vi "Set Absoulute Target Position.vi"(0 "reference in":refnum<class "SmartMotor.lvclass">, 3 "Absoulute Target Position (Revolutions)":dbl, 5 "error in (no error)":errorcluster) -> (14 "reference out":refnum<class "SmartMotor.lvclass">, 19 "error out":errorcluster)   [LabVIEW 2017, in "SmartMotor.lvclass"]
uses:
  SmartMotor.lvclass
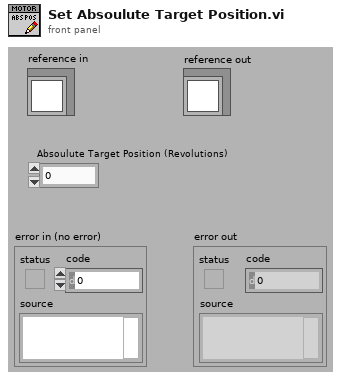
[diagram p1: front panel]
types:
  T1 = typedef "SmartMotor.lvclass/ObjectAttributes.ctl" = cluster{"SmartMotor Chain VISA Resource":refnum<visa-resource-name>, "SmartMotor Chain Address":i16, "Motor Absolute Position":i32, "Motor Relative Position":i32, "Motor Torque":i32, "Motor Voltage":i32, "Screwdriver Engaged":bool, "Screwdriver Torque Limit":i32, "Torque Monitor On/Off Status":bool, "Torque Monitor VI Reference":refnum<vi>, "Absolute Motor Torque (Filtered)":dbl, "SmartMotor Status":T2, "SmartMotor Error":T3}
  T2 = typedef "SmartMotor.lvclass/SmartMotor Status.ctl" = enum8{"Stopped", "Moving"}
  T3 = typedef "SmartMotor.lvclass/SmartMotor Error.ctl" = enum8{"None", "Read Error", "Low Voltage"}
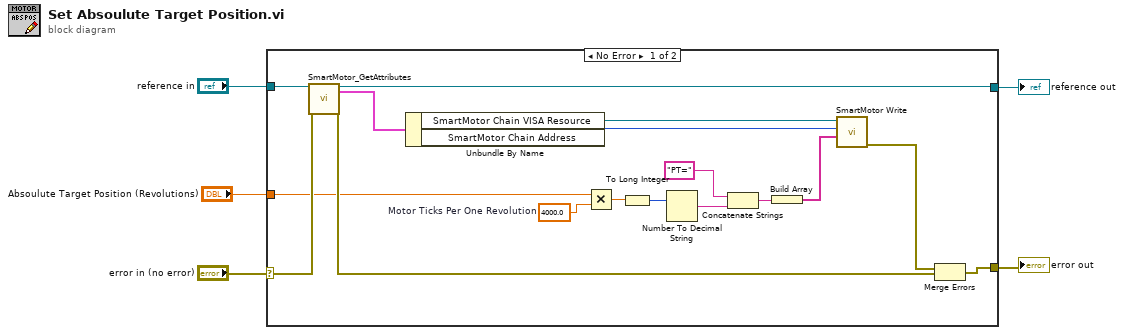
[diagram p0: block diagram]
diagram:
  n1 = case shown="No Error" "error in (no error)" {
    selector: "error in (no error)" -> [w21 w24]
    tunnel: [w19 w24] -> w4
    tunnel: [w20 w23] -> w2
    tunnel: "reference in" -> [w22 w23]
    tunnel: "Absoulute Target Position (Revolutions)" -> [w17 _]
    frame No Error {
      w15 = 4000.0  # Motor Ticks Per One Revolution
      n2 = call "SmartMotor_GetAttributes.vi"("reference in"=w22, "error in (no error)"=w21) -> ("reference out"=w20:refnum<class "SmartMotor.lvclass">, "Data"=w6:T1, "error out"=w18:errorcluster)  [unwired: 14 in, 1 out]
      n3 = Unbundle By Name(w6) -> ("SmartMotor Chain VISA Resource"=w11:refnum<visa-resource-name>, "SmartMotor Chain Address"=w7:i16)
      n4 = Multiply(x=w17, y=w15) -> (x*y=w8:dbl)
      n5 = To Long Integer(number=w8) -> (32bit integer=w9:i32)
      n6 = Number To Decimal String(number=w9) -> (decimal integer string=w13:string)  [unwired: 1 in]
      n7 = Concatenate Strings("PT=" ("string"), w13) -> (w12:string)
      n8 = Build Array(w12) -> (w10:string[])
      n9 = call "SmartMotor Write.vi"("VISA resource IN"=w11, "Motor Number"=w7, "Motor Command Array"=w10) -> ("Error Out"=w16:errorcluster)  [unwired: 4 in, 2 out]
      n10 = Merge Errors(w16, w18) -> (w19:errorcluster)
    }
    frame Error {
    }
  }
  "error out" <- w4
  "reference out" <- w2
